vi "ConvertKrakenDriveEncoders.vi"(0 "Shifter State":T1(ring), 9 "Position (Raw Sensor Units)":dbl, 11 "Velocity (Raw Sensor Units per 100 ms)":dbl, 12 "Shift Time Threshold (ms)":u32, 13 "Latched Shift Time (ms)":u32) -> (6 "Raw Velocity (rpm)":dbl, 8 "Transitioning":bool, 10 "Position (in)":dbl, 15 "Velocity (ft/s)":dbl)   [LabVIEW 2023]
doc: "This VI converts the raw Falcon 500/Talon FX encoder postion and velocity data into units of inches and feet per second, respectively. Handles low and high gear ratios."
uses:
  4f28cd8e-abc6-4562-a814-960cbb5a26e1.vi
  GlobalDrivebase.vi
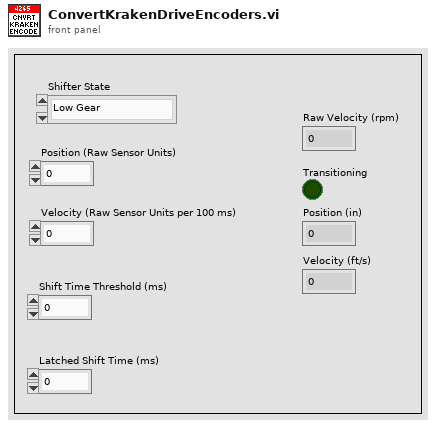
[diagram p1: front panel]
types:
  T1 = enum16{"Low Gear", "High Gear", "Transiting", "Unknown", "Force Low Gear"}
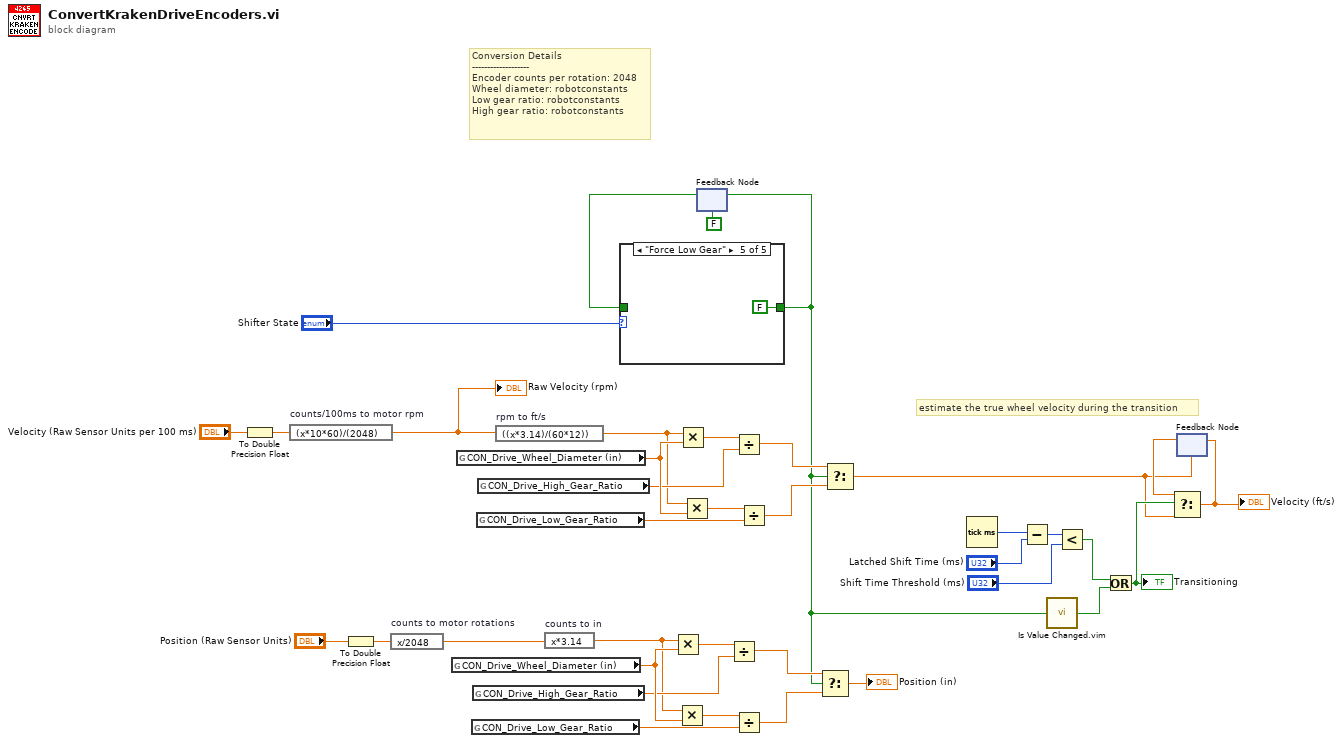
[diagram p0: block diagram]
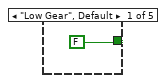
[diagram p2: hidden frame]
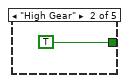
[diagram p3: hidden frame]
diagram:
  # "estimate the true wheel velocity during the transition"
  # "Conversion Details\n-------------------\nEncoder counts per rotation: 2048\nWheel diameter: robotconstants\nLow gear ratio: robotconstants\nHigh gear ratio: robotconstants"
  n1 = To Double Precision Float(number="Velocity (Raw Sensor Units per 100 ms)") -> (double precision float=w37:dbl)
  n2 = expression code="(x*10*60)/(2048)" "counts/100ms to motor rpm"(w37) -> (w35:dbl)
  "Raw Velocity (rpm)" <- w35
  n3 = To Double Precision Float(number="Position (Raw Sensor Units)") -> (double precision float=w23:dbl)
  n4 = expression code="x/2048" "counts to motor rotations"(w23) -> (w20:dbl)
  n5 = global read "GlobalDrivebase.vi" "CON_Drive_Wheel_Diameter (in)"() -> (w15:dbl)
  n6 = global read "GlobalDrivebase.vi" "CON_Drive_Wheel_Diameter (in)"() -> (w26:dbl)
  n7 = global read "GlobalDrivebase.vi" "CON_Drive_Low_Gear_Ratio"() -> (w13:dbl)
  n8 = global read "GlobalDrivebase.vi" "CON_Drive_High_Gear_Ratio"() -> (w14:dbl)
  n9 = global read "GlobalDrivebase.vi" "CON_Drive_Low_Gear_Ratio"() -> (w24:dbl)
  n10 = global read "GlobalDrivebase.vi" "CON_Drive_High_Gear_Ratio"() -> (w25:dbl)
  n11 = expression code="((x*3.14)/(60*12))" "rpm to ft/s"(w35) -> (w21:dbl)
  n12 = expression code="x*3.14" "counts to in"(w20) -> (w12:dbl)
  n13 = Multiply(x=w12, y=w15) -> (x*y=w19:dbl)
  n14 = Multiply(x=w12, y=w15) -> (x*y=w17:dbl)
  n15 = Multiply(x=w21, y=w26) -> (x*y=w30:dbl)
  n16 = Multiply(x=w21, y=w26) -> (x*y=w28:dbl)
  n17 = feedback #1(FALSE) -> (w3:bool)
  n18 = case shown="\"Force Low Gear\"" "Shifter State" {
    tunnel: [FALSE TRUE w40 w41 FALSE] -> w1
    tunnel: w3 -> [_ _ w40 w41 _]
    frame "Low Gear", Default {
    }
    frame "High Gear" {
    }
    frame "Transiting" {
    }
    frame "Unknown" {
    }
    frame "Force Low Gear" {
    }
  }
  n19 = feedback-in #1(w1) -> ()
  n20 = Divide(x=w19, y=w14) -> (x/y=w18:dbl)
  n21 = Divide(x=w30, y=w25) -> (x/y=w29:dbl)
  n22 = Divide(x=w17, y=w13) -> (x/y=w16:dbl)
  n23 = Divide(x=w28, y=w24) -> (x/y=w27:dbl)
  n24 = Select(t=w18, s=w1, f=w16) -> (s? t:f=→"Position (in)":dbl)
  n25 = Select(t=w29, s=w1, f=w27) -> (s? t:f=w5:dbl)
  n26 = Tick Count (ms)() -> (millisecond timer value=w34:u32)
  n27 = Subtract(x=w34, y="Latched Shift Time (ms)") -> (x-y=w33:u32)
  n28 = call "Is Value Changed.vim"("value"=w1) -> ("changed or first call?"=w9:bool)
  n29 = Less?(x=w33, y="Shift Time Threshold (ms)") -> (x < y?=w10:bool)
  n30 = Or(x=w10, y=w9) -> (x .or. y?=w7:bool)
  "Transitioning" <- w7
  n31 = feedback #2(w5) -> (w8:dbl)
  n32 = Select(t=w8, s=w7, f=w5) -> (s? t:f=w6:dbl)
  "Velocity (ft/s)" <- w6
  n33 = feedback-in #2(w6) -> ()
